vi "Image2ObjectsDistances2.vi"(3 "error in (no error)":errorcluster, 5 "Image Src":T2) -> (0 "error out":errorcluster, 2 "Objects bottom cords":T1(array[cluster]))   [LabVIEW 2009, in "ImageAnalysis.lvlib"]
uses:
  ImageAnalysis.lvlib
  <vilib>/vision/Image Controls.llb/IMAQ Image.ctl
  <vilib>/vision/NI_Vision_Development_Module.lvlib
  ImageProcessing.lvlib
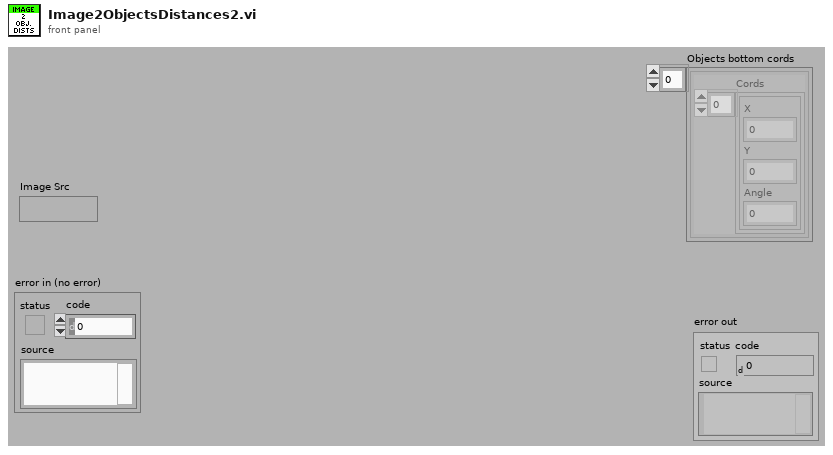
[diagram p1: front panel]
types:
  T1 = cluster{"Cords":cluster{"X":dbl, "Y":dbl, "Angle":dbl}[]}[]
  T2 = typedef "IMAQ Image.ctl" = refnum<image>
  T3 = typedef "Image Type" = u32
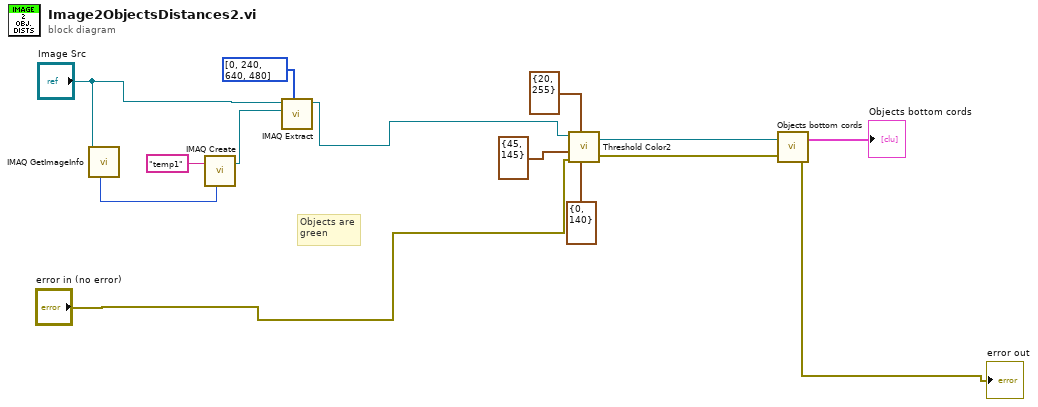
[diagram p0: block diagram]
diagram:
  # "Objects are\ngreen"
  n1 = call "IMAQ GetImageInfo"("Image"="Image Src") -> ("Image Type"=w8:T3)  [unwired: 3 in, 7 out]
  n2 = call "IMAQ Create"("Image Name"="temp1", "Image Type"=w8) -> ("New Image"=w10:T2)  [unwired: 3 in, 1 out]
  n3 = call "IMAQ Extract"("Optional Rectangle"=i32[] [0, 240, 640, 480], "Image Dst"=w10, "Image Src"="Image Src") -> ("Image Dst Out"=w5:T2)  [unwired: 7 in, 1 out]
  n4 = call "Threshold Color2.vi"("Luma Range"=cluster{"Lower value":i32, "Upper value":i32} {"Lower value"=0, "Upper value"=140} ("Val or Inten Range"), "Sat Range"=cluster{"Lower value":i32, "Upper value":i32} {"Lower value"=20, "Upper value"=255}, "error in (no error)"="error in (no error)", "Hue Range"=cluster{"Lower value":i32, "Upper value":i32} {"Lower value"=45, "Upper value"=145}, "Image Src"=w5) -> ("error out"=w13:errorcluster, "Image Dst Out"=w1:T2)  [unwired: 1 in]
  n5 = call "Objects bottom cords.vi"("error in (no error)"=w13, "Image"=w1) -> ("error out"=→"error out":errorcluster, "Objects bottom cords"=→"Objects bottom cords":T1)
